vi "getCallerVIname.vi"() -> (17 "VI name":string)   [LabVIEW 2012]
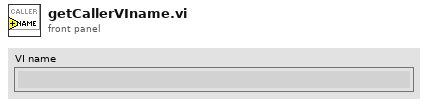
[diagram p1: front panel]
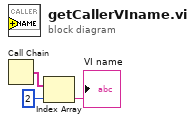
[diagram p0: block diagram]
diagram:
  n1 = Call Chain() -> (call chain=w3:string[])
  n2 = Index Array(array=w3, index=2) -> (element=→"VI name":string)
